vi "Derate&MI.vi"(0 "Frequency (MHz)":dbl format="%.2f", 1 "neg peak pressure (MPa)":dbl format="%.2f", 2 "Intensity Variables":T2 {"Pulse Int \nIntegral (PII J/cm^2)" format="%.4e"; "Pulse Av Intensity\n (Ipa W/cm^2)" format="%.2f"; "Temporal Av Intensity \n(Ita mW/cm^2)" format="%.2f"; "pulse dur (Pd s)" format="%.2e"}, 3 "pos peak pressure (MPa)":dbl format="%.2f", 4 "delay (ms)":dbl format="%.2f", 5 "prf":dbl format="%.2f") -> (7 "Pulse Parameters":T1 {"pos peak pressure (MPa)" format="%.2f"; "focal length (cm)" format="%.2f"; "MI" format="%.2f"; "Ita.3" format="%.2f"; "Temporal Av Intensity \n(Ita mW/cm^2)" format="%.2f"; "Ipa.3" format="%.2f"; "Pulse Av Intensity\n (Ipa W/cm^2)" format="%.2f"; "Pulse Int \nIntegral (PII J/cm^2)" format="%.4e"; "pulse dur (Pd s)" format="%.2e"; "p.3" format="%.2e"; "neg peak pressure (MPa)" format="%.2f"; "derating (.3) factor" format="%.2f"; "prf" format="%.2f"; "Frequency (MHz)" format="%.2f"})   [LabVIEW 2022 SP3]
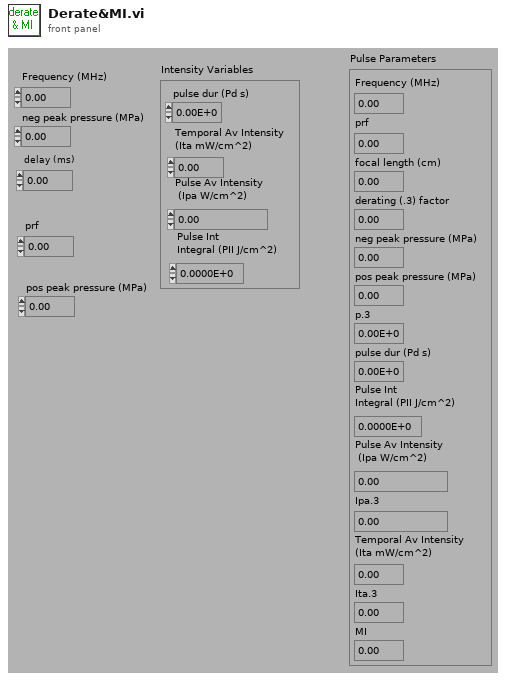
[diagram p1: front panel]
types:
  T1 = cluster{"Frequency (MHz)":dbl, "prf":dbl, "focal length (cm)":dbl, "derating (.3) factor":dbl, "neg peak pressure (MPa)":dbl, "pos peak pressure (MPa)":dbl, "p.3":dbl, "pulse dur (Pd s)":dbl, "Pulse Int \nIntegral (PII J/cm^2)":dbl, "Pulse Av Intensity\n (Ipa W/cm^2)":dbl, "Ipa.3":dbl, "Temporal Av Intensity \n(Ita mW/cm^2)":dbl, "Ita.3":dbl, "MI":dbl}
  T2 = cluster{"pulse dur (Pd s)":dbl, "Temporal Av Intensity \n(Ita mW/cm^2)":dbl, "Pulse Av Intensity\n (Ipa W/cm^2)":dbl, "Pulse Int \nIntegral (PII J/cm^2)":dbl}
  T3 = cluster{"Frequency (MHz)":dbl, "prf":dbl, dbl, dbl, "neg peak pressure (MPa)":dbl, "pos peak pressure (MPa)":dbl, dbl, "pulse dur (Pd s)":dbl, "Pulse Int \nIntegral (PII J/cm^2)":dbl, "Pulse Av Intensity\n (Ipa W/cm^2)":dbl, dbl, "Temporal Av Intensity \n(Ita mW/cm^2)":dbl, dbl, dbl}
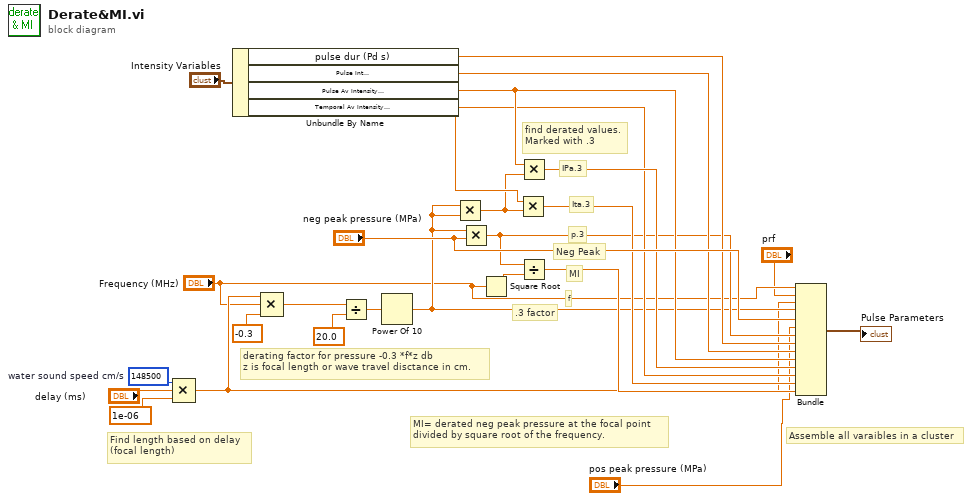
[diagram p0: block diagram]
diagram:
  w20 = 148500  # water sound speed cm/s
  # "MI= derated neg peak pressure at the focal point\ndivided by square root of the frequency."
  # "Find length based on delay\n(focal length)"
  # "f"
  # "p.3"
  # "Neg Peak"
  # "MI"
  # ".3 factor"
  # "IPa.3"
  # "Ita.3"
  # "Assemble all varaibles in a cluster"
  # "find derated values.\nMarked with .3"
  # "derating factor for pressure -0.3 *f*z db\nz is focal length or wave travel disctance in cm."
  n1 = Compound Arithmetic op=MULTIPLY(w20, "delay (ms)", 1e-06 ("x")) -> (w4:dbl)
  n2 = Unbundle By Name("Intensity Variables") -> ("pulse dur (Pd s)"=w15:dbl, "Pulse Int \nIntegral (PII J/cm^2)"=w14:dbl, "Pulse Av Intensity\n (Ipa W/cm^2)"=w13:dbl, "Temporal Av Intensity \n(Ita mW/cm^2)"=w10:dbl)
  n3 = Compound Arithmetic op=MULTIPLY(w4, "Frequency (MHz)", -0.3 ("x")) -> (w18:dbl)
  n4 = Divide(x=w18, y=20.0) -> (x/y=w23:dbl)
  n5 = Power Of 10(x=w23) -> (10^x=w5:dbl)
  n6 = Multiply(x=w5, y=w5) -> (x*y=w7:dbl)
  n7 = Multiply(x=w5, y="neg peak pressure (MPa)") -> (x*y=w6:dbl)
  n8 = Square Root(x="Frequency (MHz)") -> (sqrt(x)=w21:dbl)
  n9 = Multiply(x=w10, y=w7) -> (x*y=w9:dbl)
  n10 = Multiply(x=w13, y=w7) -> (x*y=w12:dbl)
  n11 = Divide(x=w6, y=w21) -> (x/y=w8:dbl)
  n12 = Bundle("Frequency (MHz)"="Frequency (MHz)", "prf"="prf", w4, w5, "neg peak pressure (MPa)"="neg peak pressure (MPa)", "pos peak pressure (MPa)"="pos peak pressure (MPa)", w6, "pulse dur (Pd s)"=w15, "Pulse Int \nIntegral (PII J/cm^2)"=w14, "Pulse Av Intensity\n (Ipa W/cm^2)"=w13, w12, "Temporal Av Intensity \n(Ita mW/cm^2)"=w10, w9, w8) -> (→"Pulse Parameters":T3)  [unwired: 1 out]
